vi "A3 GPS Decoding.vi"() -> ()   [LabVIEW 2018]
uses:
  <vilib>/Utility/file.llb/Write Delimited Spreadsheet (string).vi
panel:
  in  "file path (dialog if empty)":path
  in  "error in":errorcluster
  out "error out":errorcluster
  in  "file path (use dialog)":path
  out "Data Table":string[][](table)
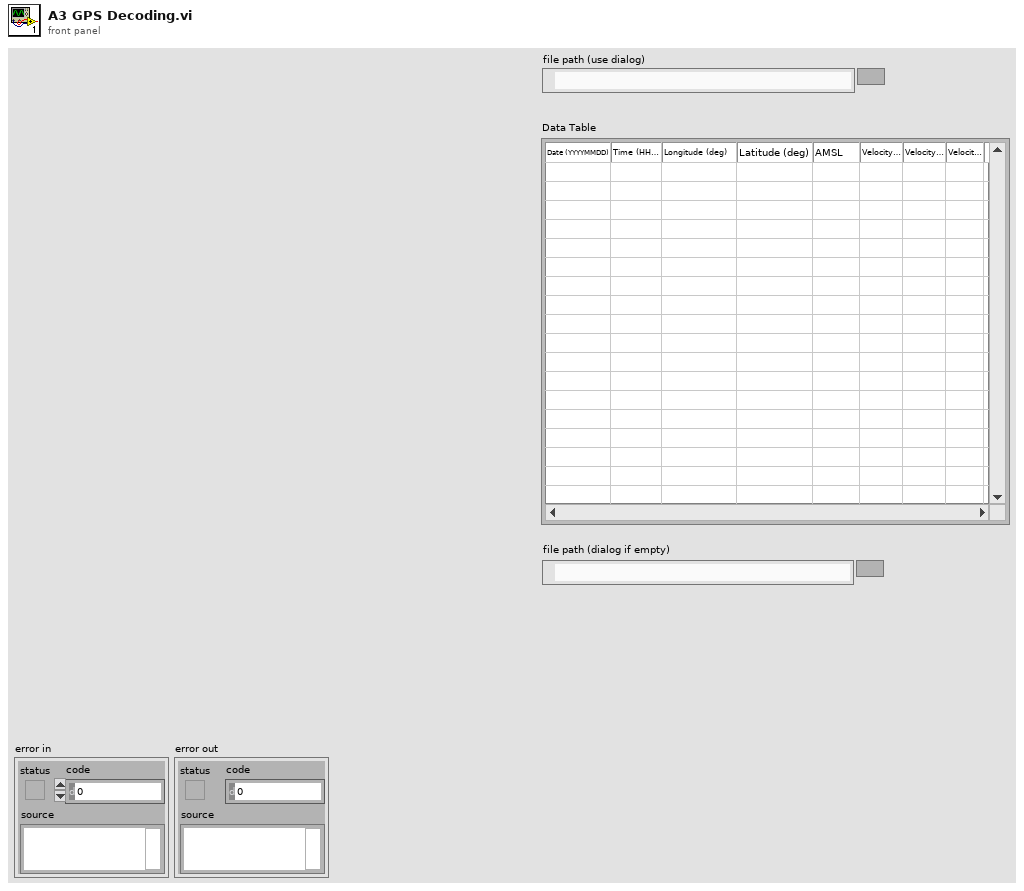
[diagram p1: front panel]
types:
  T1 = enum16{"open", "replace", "create", "open or create", "replace or create", "replace or create with confirmation"}
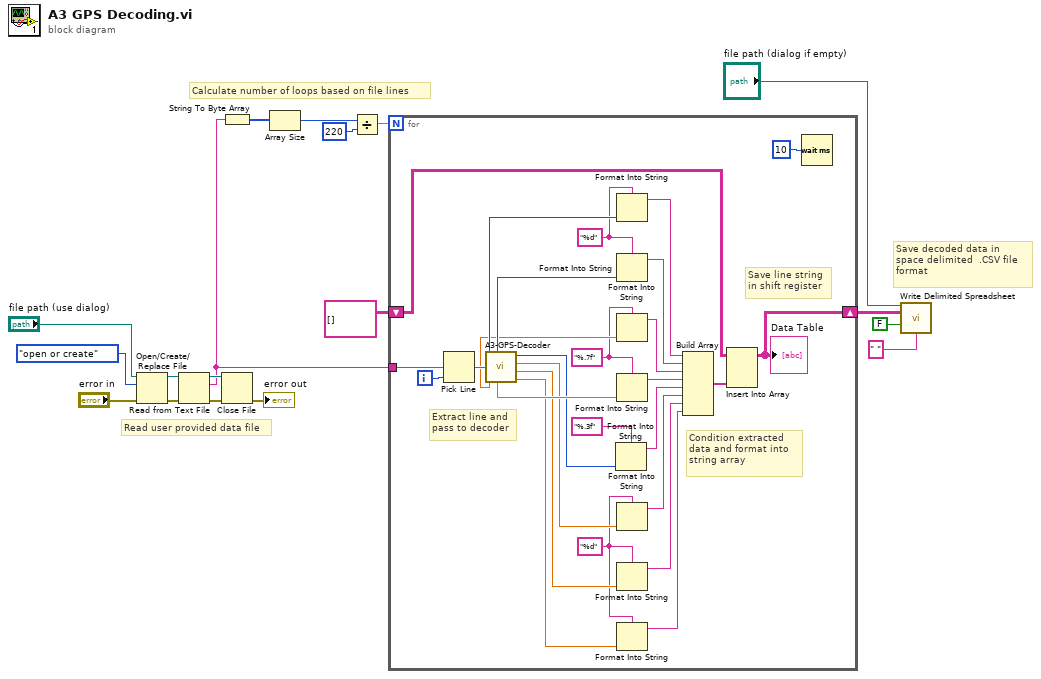
[diagram p0: block diagram]
diagram:
  # "Save decoded data in \nspace delimited  .CSV file \nformat"
  # "Calculate number of loops based on file lines"
  # "Read user provided data file"
  n1 = Open/Create/Replace File(file path (use dialog)="file path (use dialog)", error in="error in", operation (0:open)=T1."open or create") -> (refnum out=w17:refnum<file>, error out=w16:errorcluster)  [unwired: 3 in, 1 out]
  n2 = Read from Text File(file (use dialog)=w17, error in=w16) -> (refnum out=w12:refnum<file>, text=w9:string, error out=w13:errorcluster)  [unwired: 2 in, 1 out]
  n3 = String To Byte Array(string=w9) -> (unsigned byte array=w8:u8[])
  n4 = Close File(refnum=w12, error in=w13) -> (error out=→"error out":errorcluster)  [unwired: 1 out]
  n5 = Array Size(array=w8) -> (size(s)=w7:i32)
  n6 = Divide(x=w7, y=220) -> (x/y=w5:dbl)
  n7 = for {
    N: w5 -> [_]
    tunnel: w9 -> [w44]
    shift-right: [w33] -> w2
    shift-left: string[][] [] -> [w43]
    i -> [w45]
    w19 = "%d" ("format string")
    w21 = "%.7f" ("format string")
    w22 = "%d" ("format string")
    # "Save line string \nin shift register"
    # "Condition extracted\ndata and format into \nstring array"
    # "Extract line and\npass to decoder"
    n8 = Pick Line(multi-line string=w44, line index=w45) -> (output string=w31:string)  [unwired: 1 in]
    n9 = call "A3-GPS-Decoder.vi"("ASCII Hexidecimal String"=w31) -> ("Date (YYYYMMDD)"=w30:u32, "Time (HHMMSS)"=w29:u32, "Longitude (Deg)"=w28:dbl, "Latitude (Deg)"=w27:dbl, "AMSL (m)"=w26:u32, "Velocity North (cm/s)"=w25:sgl, "Velocity East (cm/s)"=w24:sgl, "Velocity Down (cm/s)"=w23:sgl)
    n10 = Format Into String(format string="%.3f", w26) -> (resulting string=w39:string)  [unwired: 2 in, 1 out]
    n11 = Format Into String(format string=w22, w30) -> (resulting string=w34:string)  [unwired: 2 in, 1 out]
    n12 = Format Into String(format string=w22, w29) -> (resulting string=w42:string)  [unwired: 2 in, 1 out]
    n13 = Format Into String(format string=w21, w28) -> (resulting string=w41:string)  [unwired: 2 in, 1 out]
    n14 = Format Into String(format string=w21, w27) -> (resulting string=w40:string)  [unwired: 2 in, 1 out]
    n15 = Format Into String(format string=w19, w25) -> (resulting string=w38:string)  [unwired: 2 in, 1 out]
    n16 = Format Into String(format string=w19, w24) -> (resulting string=w37:string)  [unwired: 2 in, 1 out]
    n17 = Format Into String(format string=w19, w23) -> (resulting string=w36:string)  [unwired: 2 in, 1 out]
    n18 = Build Array(w34, w42, w41, w40, w39, w38, w37, w36) -> (w35:string[])
    n19 = Insert Into Array(array=w43, new element=w35) -> (w33:string[][])  [unwired: 2 in]
    "Data Table" <- w33
    n20 = Wait (ms)(milliseconds to wait=u32 10) -> ()  [unwired: 1 out]
  }
  n21 = call-poly <vilib>:"Write Delimited Spreadsheet.vi"("file path (dialog if empty)"="file path (dialog if empty)", "2D data"=w2, "append to file? (new file:F)"=FALSE, "delimiter (\\t)"=" " ("delimiter (\\t)")) -> ()  [unwired: 10 in, 2 out]
